vi "ReadConsecutiveFrames.vi"(9 "STP Loop Data In":T1, 10 "CAN Data":T2[](array[typedef]) {"payload" format="%x"; "timestamp" format="%<%.7X\n%x>T"; "type" items=["CAN Data"=0, "CAN Remote"=1, "CAN Bus Error"=2, "CAN 2.0 Data"=8, "CAN FD Data"=16, "CAN FD+BRS Data"=24, "J1939 Data"=192, "Delay"=224, "Log Trigger"=225, "Start Trigger"=226]; "identifier" format="%x"}, 11 "RxID":u32=2043 format="%x") -> (1 "STP Loop Data Out":T1)   [LabVIEW 2023, in "HardwareAbstractionLayer_LVOOP.lvlib" / "CAN Application Protocols Lib.lvlib" / "STP Protocol.lvclass"]
uses:
  STP Protocol.lvclass
  <vilib>/xnet/xnet.llb/XNET Frame CAN.ctl
  <vilib>/xnet/xnet.llb/XNET Frame Type CAN.ctl
  Ctrls/STP Loop Data.ctl
  Ctrls/TP Frame Type.ctl
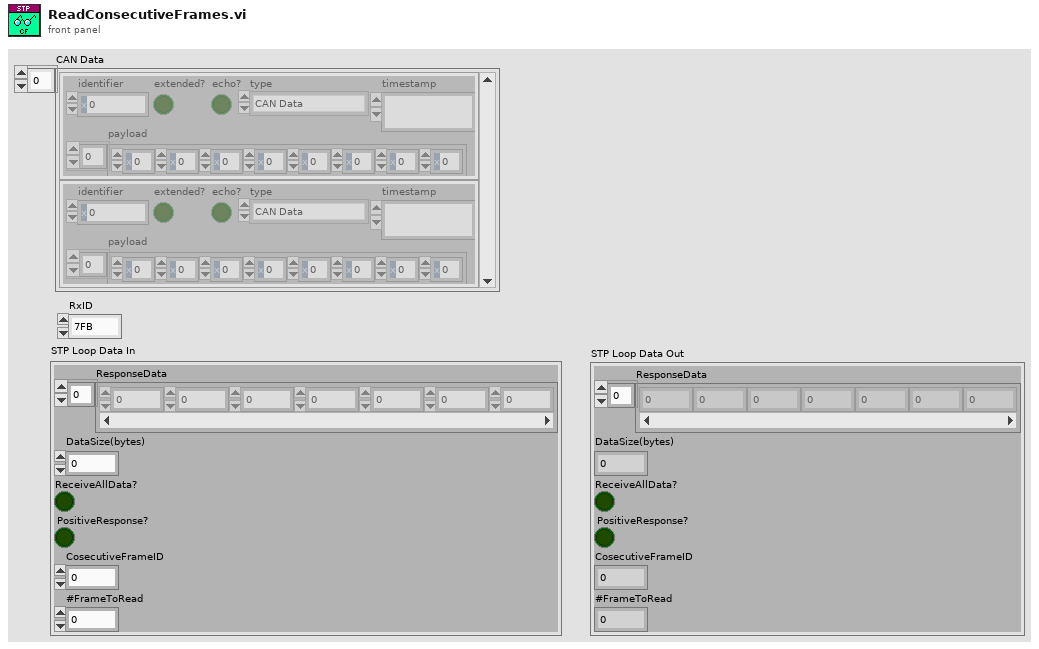
[diagram p1: front panel]
types:
  T1 = typedef "HardwareAbstractionLayer_LVOOP.lvlib/CAN Application Protocols Lib.lvlib/STP Protocol.lvclass/STP Loop Data.ctl" = cluster{"ResponseData":u8[], "DataSize(bytes)":u16, "ReceiveAllData?":bool, "PositiveResponse?":bool, "CosecutiveFrameID":fxp<+,4,4>, "#FrameToRead":i32}
  T2 = typedef "XNET Frame CAN.ctl" = cluster{"timestamp":timestamp, "payload":u8[], "identifier":u32, "type":T3, "extended?":bool, "echo?":bool}
  T3 = typedef "XNET Frame Type CAN.ctl" = u8
  T4 = typedef "HardwareAbstractionLayer_LVOOP.lvlib/CAN Application Protocols Lib.lvlib/STP Protocol.lvclass/TP Frame Type.ctl" = u8
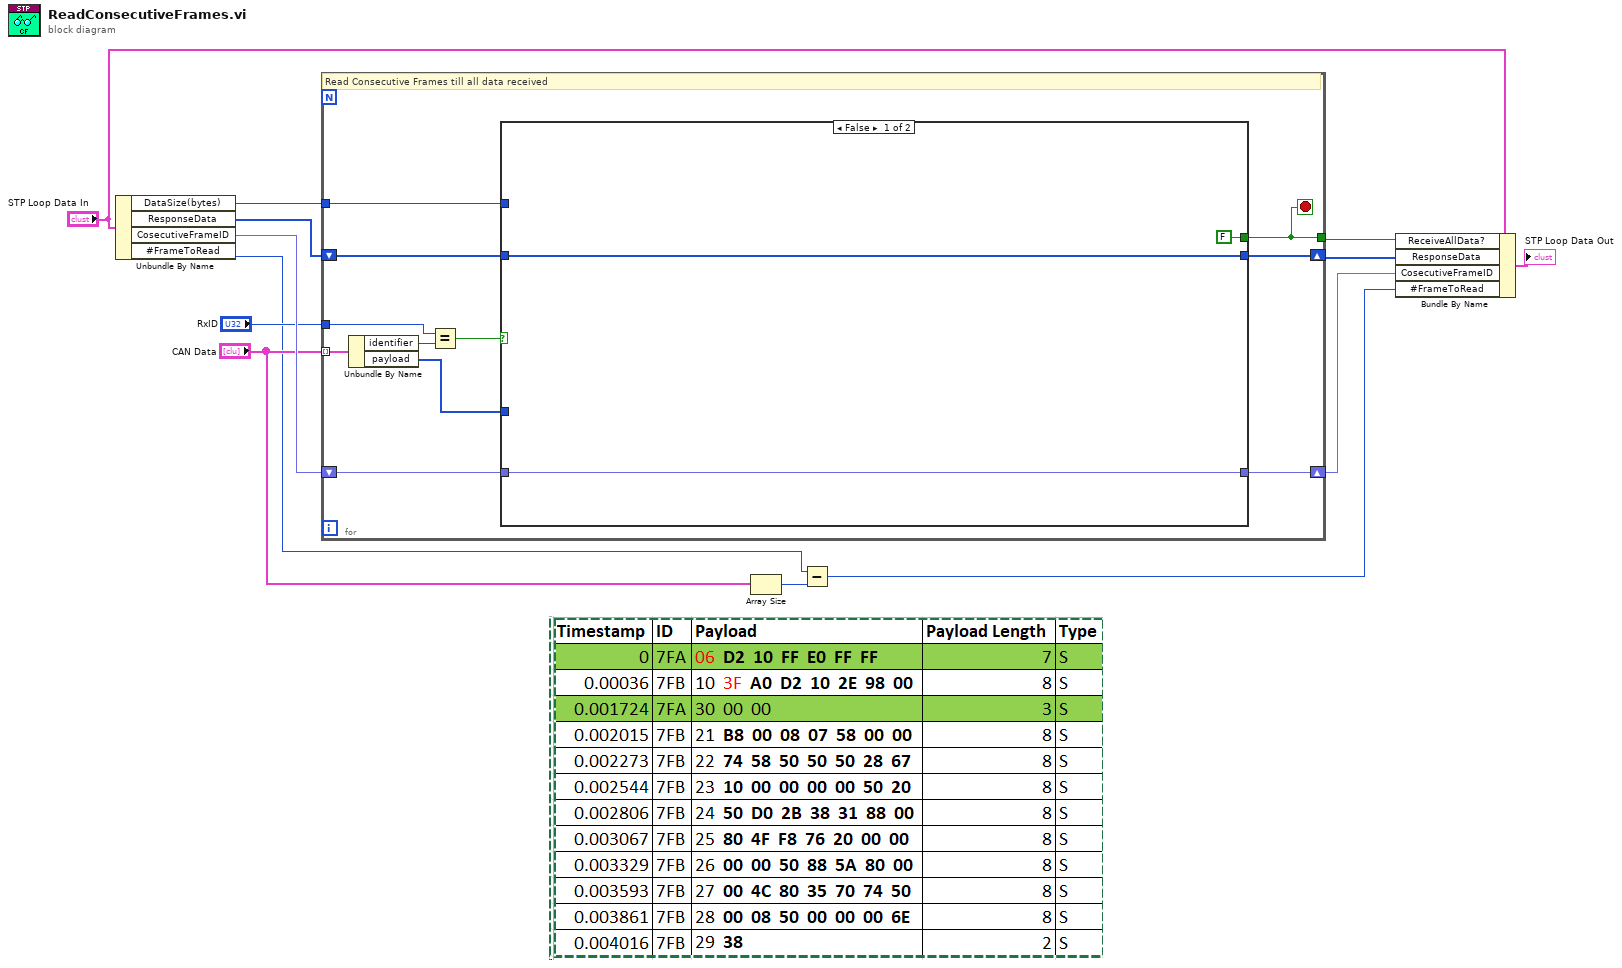
[diagram p0: block diagram]
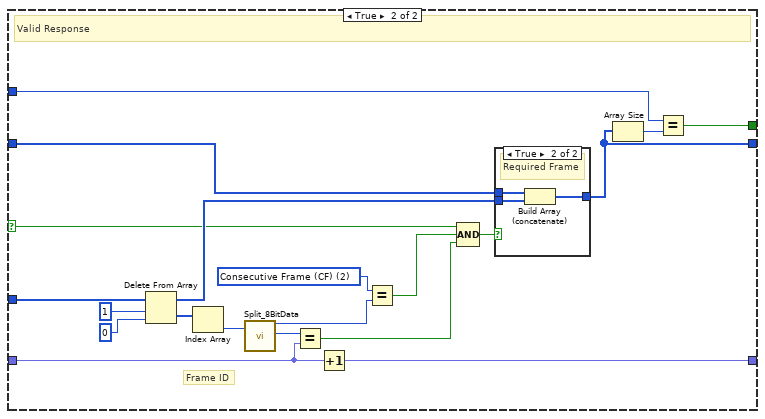
[diagram p2: hidden frame]
diagram:
  n1 = Unbundle By Name("STP Loop Data In") -> ("DataSize(bytes)"=w13:u16, "ResponseData"=w12:u8[], "CosecutiveFrameID"=w11:fxp<+,4,4>, "#FrameToRead"=w2:i32)
  n2 = for {
    tunnel: "CAN Data" -> [w24] mode=indexing
    shift-right: [w17] -> w8
    shift-left: w12 -> [w21]
    shift-right: [w18] -> w6
    shift-left: w11 -> [w19]
    tunnel: w13 -> [w16]
    tunnel: [w15] -> w7
    tunnel: "RxID" -> [w14]
    stop <- w15 stop-if-true
    # "Read Consecutive Frames till all data received"
    n3 = Unbundle By Name(w24) -> ("identifier"=w23:u32, "payload"=w22:u8[])
    n4 = Equal?(x=w14, y=w23) -> (x = y?=w20:bool)
    n5 = case shown="False" w20 {
      selector: w20 -> [_ w42]
      tunnel: w22 -> [_ w47]
      tunnel: w21 -> [w26 w43]
      tunnel: w19 -> [w25 w40]
      tunnel: [w25 w39] -> w18
      tunnel: [w26 w37] -> w17
      tunnel: w16 -> [_ w35]
      tunnel: [FALSE w34] -> w15
      frame False {
      }
      frame True {
        w31 = T4 2 items=["Single Frame (SF)", "First Frame (SF)", "Consecutive Frame (CF)", "Flow Control Frame (FC)"] ("Ring")
        # "Frame ID"
        # "Valid Response"
        n6 = Delete From Array(array=w47, length=1, index=0) -> (deleted portion=w41:u8[], array with subset deleted=w44:u8[])
        n7 = Index Array(array=w41) -> (element=w33:u8)  [unwired: 1 in]
        n8 = call "Split_8BitData.vi"("x"=w33) -> ("hi(x)"=w30:u8, "lo(x)"=w32:u8)  [unwired: 17 in]
        n9 = Equal?(x=w32, y=w40) -> (x = y?=w28:bool)
        n10 = Increment(x=w40) -> (x+1=w39:fxp<+,4,4>)
        n11 = Equal?(x=w31, y=w30) -> (x = y?=w29:bool)
        n12 = Compound Arithmetic op=AND(w42, w29, w28) -> (w38:bool)
        n13 = case shown="True" w38 {
          tunnel: w44 -> [_ w51]
          tunnel: w43 -> [w48 w50]
          tunnel: [w48 w49] -> w37
          frame False {
          }
          frame True {
            # "Required Frame"
            n14 = Build Array (concatenate)(w50, w51) -> (w49:u8[])
          }
        }
        n15 = Array Size(array=w37) -> (size(s)=w36:i32)
        n16 = Equal?(x=w35, y=w36) -> (x = y?=w34:bool)
      }
    }
  }
  n17 = Array Size(array="CAN Data") -> (size(s)=w4:i32)
  n18 = Subtract(x=w2, y=w4) -> (x-y=w1:i32)
  n19 = Bundle By Name(cluster="STP Loop Data In", "ReceiveAllData?"=w7, "ResponseData"=w8, "CosecutiveFrameID"=w6, "#FrameToRead"=w1) -> (→"STP Loop Data Out":T1)
